vi "UDP 클라02.vi"() -> ()   [LabVIEW 2018]
uses:
  <vilib>/Utility/tcp.llb/UDP Multicast Read-Only Open.vi
panel:
  out "데이터 출력":string
  in  "정지":bool
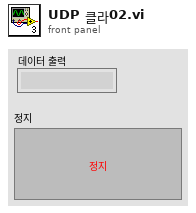
[diagram p1: front panel]
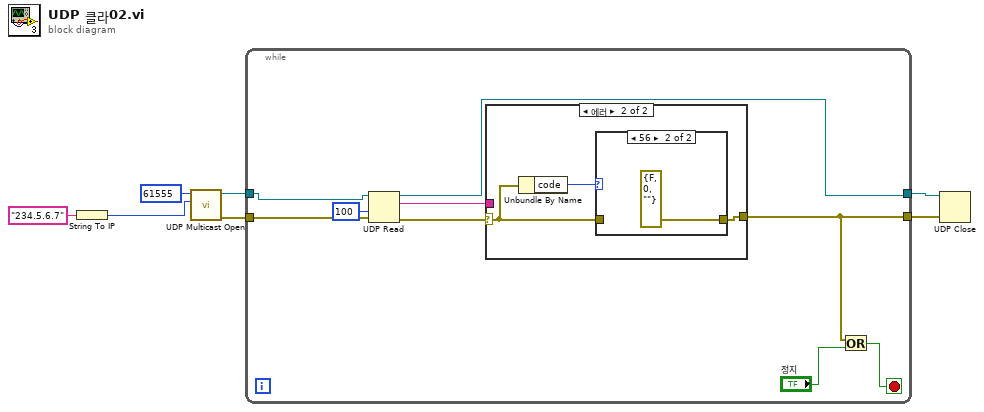
[diagram p0: block diagram]
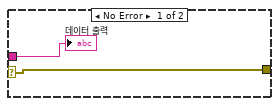
[diagram p2: hidden frame]
diagram:
  n1 = String To IP(1:"234.5.6.7" ("이름")) -> (0:w1:u32)
  n2 = call-poly <vilib>:"UDP Multicast Open.vi"("multicast addr"=w1, "port"=u16 61555 ("포트")) -> ("error out"=w5:errorcluster, "connection ID"=w7:refnum<k16>)  [unwired: 7 in, 1 out]
  n3 = while {
    tunnel: w7 -> [w11]
    tunnel: [w10] -> w6
    tunnel: w5 -> [w16]
    tunnel: [w12] -> w4
    stop <- w14 stop-if-true
    n4 = UDP Read(connection ID=w11, timeout ms (25000)=100 ("타임아웃 ms (25000)"), 8:w16) -> (data out=w9:string, error out=w13:errorcluster, 3:w10:refnum<k16>)  [unwired: 1 in, 2 out]
    n5 = case shown="에러" w13 {
      selector: w13 -> [w18 w19]
      tunnel: [w18 w20] -> w12
      tunnel: w9 -> [w17 _]
      frame No Error {
        "데이터 출력" <- w17
      }
      frame Error {
        n6 = Unbundle By Name(w19) -> ("code"=w21:i32)
        n7 = case shown="56" w21 {
          tunnel: [w22 errorcluster {"status"=FALSE, "code"=0, "source"=""} ("에러 상수")] -> w20
          tunnel: w19 -> [w22 _]
          frame Default {
          }
          frame 56 {
          }
        }
      }
    }
    n8 = Or(x=w12, y="정지") -> (x .or. y?=w14:bool)
  }
  n9 = UDP Close(connection ID=w6, 8:w4) -> ()  [unwired: 2 out]
